vi "Subtract Rational Polynomials.vi"   [LabVIEW 2018, in "NI_AALPro.lvlib"]
doc: "Subtracts rational polynomial G2 from rational polynomial G1. The data types you wire to the <B>Numerator 1</B>, <B>Denominator 1</B>, <B>Numerator 2</B>, and <B>Denominator 2</B> inputs determine the polymorphic instance to use."
uses:
  <vilib>/Analysis/NI_AALPro.lvlib
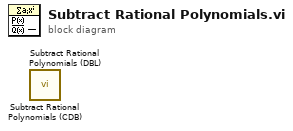
[diagram p0: block diagram]
diagram:
  n1 = call "Subtract Rational Polynomials (CDB).vi"() -> ()  [unwired: 9 in, 3 out]
  n2 = call "Subtract Rational Polynomials (DBL).vi"() -> ()  [unwired: 9 in, 3 out]
